vi "ReadWriteREPL.vi"(7 "Wait?":bool=TRUE, 8 "error in":errorcluster, 9 "Console In":string, 10 "write buffer":string, 11 "VISA in":refnum<visa-resource-name>) -> (0 "error out":errorcluster, 1 "Console Out":string, 2 "Update?":bool, 3 "VISA out":refnum<visa-resource-name>, 5 "new text":string)   [LabVIEW 2016]
panel:
  out "Array":string[](array[string])
  # "T = Send cmd (s)/wait for reply\nF = send a char and grab the buffer"
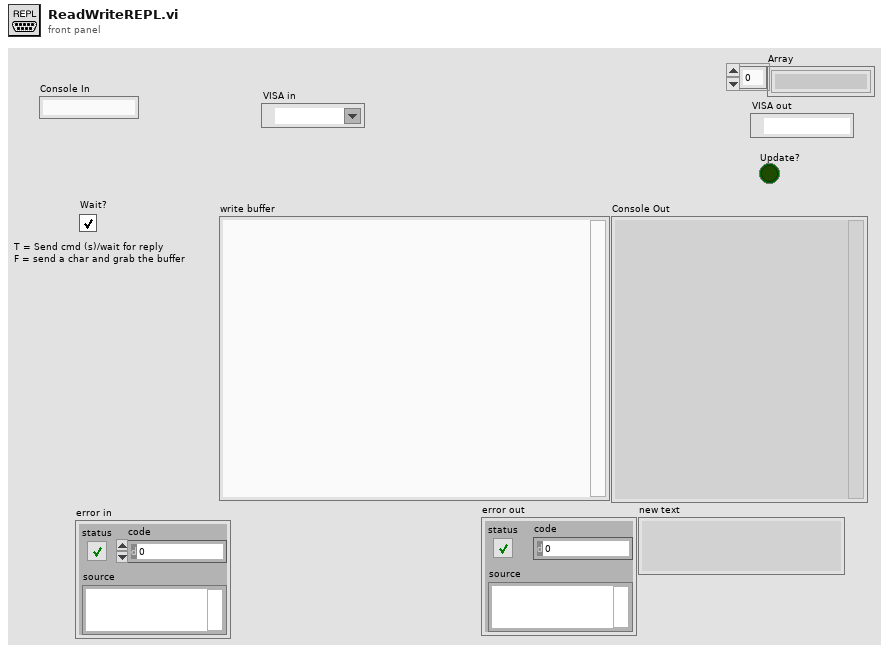
[diagram p1: front panel]
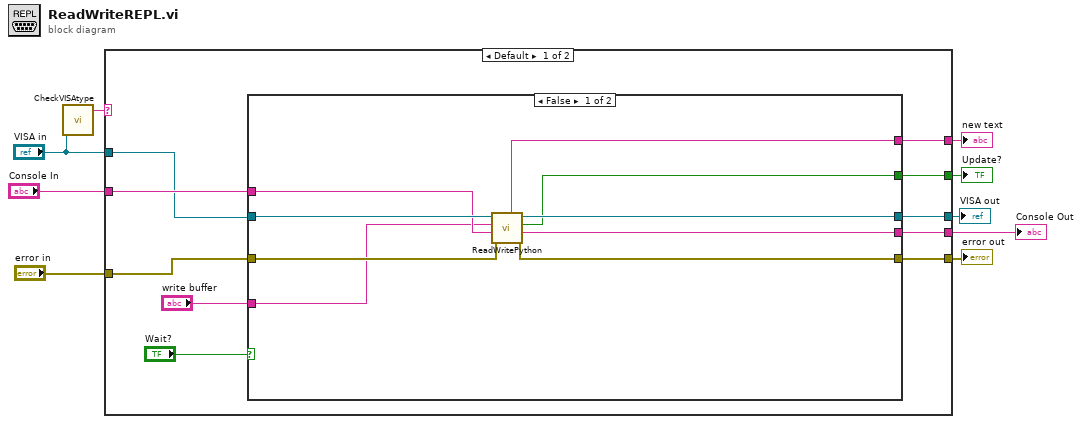
[diagram p0: block diagram]
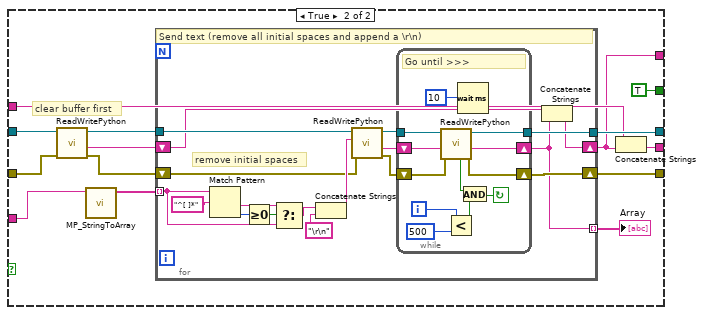
[diagram p2: hidden frame]
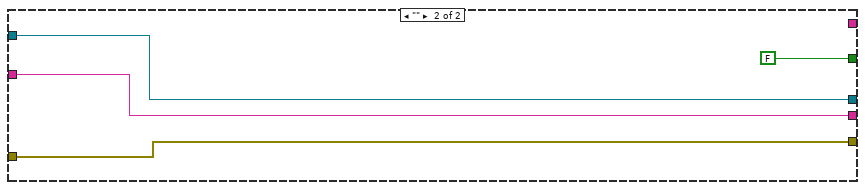
[diagram p3: hidden frame]
diagram:
  n1 = call "CheckVISAtype.vi"("VISA Refnum in"="VISA in") -> ("data string"=w1:string)  [unwired: 9 in, 1 out]
  n2 = case shown="Default" w1 {
    tunnel: "VISA in" -> [w10 w76]
    tunnel: "error in" -> [w11 w74]
    tunnel: "Console In" -> [w17 w75]
    tunnel: [w16 w76] -> w7
    tunnel: [w15 w75] -> w6
    tunnel: [w14 w74] -> w5
    tunnel: [w13 FALSE ("Update?")] -> w4
    tunnel: [w12 _] -> w3
    frame Default {
      n3 = case shown="False" "Wait?" {
        tunnel: w10 -> [w27 w38]
        tunnel: w17 -> [w24 w31]
        tunnel: w11 -> [w28 w36]
        tunnel: "write buffer" -> [w22 w34]
        tunnel: [w26 w41] -> w16
        tunnel: [w23 w29] -> w15
        tunnel: [w25 w40] -> w14
        tunnel: [w21 TRUE ("Update?")] -> w13
        tunnel: [w20 w30] -> w12
        frame False {
          n4 = call "ReadWritePython.vi"("error in"=w28, "Console In"=w24, "Write"=w22, "VISA in"=w27) -> ("error out"=w25:errorcluster, "Console Out"=w23:string, "Update?"=w21:bool, "VISA out"=w26:refnum<visa-resource-name>, "read buffer"=w20:string)  [unwired: 2 in, 1 out]
        }
        frame True {
          # "clear buffer first"
          n5 = call "ReadWritePython.vi"("error in"=w36, "VISA in"=w38) -> ("error out"=w35:errorcluster, "Console Out"=w33:string, "VISA out"=w37:refnum<visa-resource-name>)  [unwired: 4 in, 3 out]
          n6 = call "MP_StringToArray.vi"("write buffer"=w34) -> ("Array"=w42:string[])  [unwired: 10 in]
          n7 = for {
            tunnel: w37 -> [w60]
            tunnel: w42 -> [w52] mode=indexing
            shift-right: [w43] -> w30
            shift-left: w33 -> [w45]
            shift-right: [w46] -> w40
            shift-left: w35 -> [w57]
            tunnel: [w48] -> w41
            tunnel: [w44] -> w32 mode=indexing
            # "remove initial spaces"
            # "Send text (remove all initial spaces and append a \\r\\n)"
            n8 = Match Pattern(string=w52, regular expression="^[ ]*") -> (after substring=w53:string, offset past match=w55:i32)  [unwired: 1 in, 2 out]
            n9 = Greater Or Equal To 0?(x=w55) -> (x >= 0?=w54:bool)
            n10 = Select(t=w53, s=w54, f=w52) -> (s? t:f=w51:string)
            n11 = Concatenate Strings(w51, "\r\n" ("write buffer")) -> (w59:string)
            n12 = call "ReadWritePython.vi"("error in"=w57, "Write"=w59, "VISA in"=w60) -> ("error out"=w49:errorcluster, "Console Out"=w47:string, "VISA out"=w50:refnum<visa-resource-name>)  [unwired: 3 in, 3 out]
            n13 = while {
              tunnel: w50 -> [w72]
              tunnel: [w71] -> w48
              shift-right: [w69] -> w44
              shift-left: w47 -> [w70]
              shift-right: [w67] -> w46
              shift-left: w49 -> [w68]
              i -> [w65]
              stop <- w63 continue-if-true
              # "Go until >>>"
              n14 = call "ReadWritePython.vi"("error in"=w68, "Console In"=w70, "VISA in"=w72) -> ("error out"=w67:errorcluster, "Console Out"=w69:string, "VISA out"=w71:refnum<visa-resource-name>, "Not Done?"=w62:bool)  [unwired: 3 in, 2 out]
              n15 = Less?(x=w65, y=500) -> (x < y?=w61:bool)
              n16 = Wait (ms)(milliseconds to wait=u32 10) -> ()  [unwired: 1 out]
              n17 = And(x=w62, y=w61) -> (x .and. y?=w63:bool)
            }
            n18 = Concatenate Strings(w45, w44) -> (w43:string)
          }
          "Array" <- w32
          n19 = Concatenate Strings(w31, w30) -> (w29:string)
        }
      }
    }
    frame "" {
    }
  }
  "Console Out" <- w6
  "VISA out" <- w7
  "error out" <- w5
  "Update?" <- w4
  "new text" <- w3
